vi "Create Event.vi"(3 "error in (no error)":errorcluster, 4 "ExecAnchor in":refnum<class "ExecAnchor.lvclass">) -> (0 "error out":errorcluster, 1 "Event Reg":refnum<event-registration>)   [LabVIEW 2020, in "ExecAnchor.lvclass"]
uses:
  ExecAnchor.lvclass
  ExecAnchor.lvclass/ExecAnchor.ctl
  <vilib>/Utility/error.llb/Error Cluster From Error Code.vi
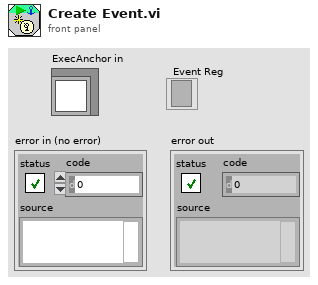
[diagram p1: front panel]
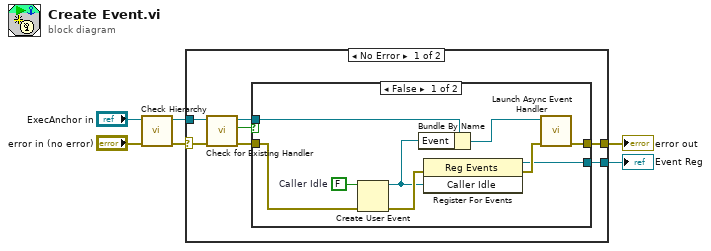
[diagram p0: block diagram]
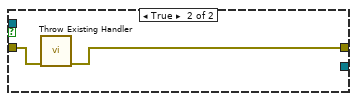
[diagram p2: hidden frame]
diagram:
  n1 = call "Check Hierarchy.vi"("error in (no error)"="error in (no error)", "ExecAnchor in"="ExecAnchor in") -> ("error out"=w2:errorcluster, "ExecAnchor out"=w4:refnum<class "ExecAnchor.lvclass">)  [unwired: 8 in]
  n2 = case shown="No Error" w2 {
    selector: w2 -> [w10 w25]
    tunnel: [w12 _] -> w5
    tunnel: w4 -> [w11 _]
    tunnel: [w13 w25] -> w1
    frame No Error {
      n3 = call "Check for Existing Handler.vi"("error in (no error)"=w10, "ExecAnchor in"=w11) -> ("error out"=w9:errorcluster, "Existing Handler"=w7:bool, "ExecAnchor out"=w8:refnum<class "ExecAnchor.lvclass">)  [unwired: 7 in]
      n4 = case shown="False" w7 {
        tunnel: [w15 w23] -> w13
        tunnel: [w18 _] -> w12
        tunnel: w8 -> [w17 _]
        tunnel: w9 -> [w16 w24]
        frame False {
          w20 = FALSE  # Caller Idle
          n5 = Create User Event(user event datatype=w20, error in=w16) -> (user event=w19:refnum<user-event>, error out=w21:errorcluster)
          n6 = Bundle By Name(cluster=w17, "Event"=w19) -> (w14:refnum<class "ExecAnchor.lvclass">)
          n7 = register-events(error in=w21, w19) -> (reference out=w18:refnum<event-registration>, error out=w22:errorcluster)  [unwired: 1 in]
          n8 = call "Launch Async Event Handler.vi"("error in (no error)"=w22, "ExecAnchor in"=w14) -> ("error out"=w15:errorcluster)  [unwired: 8 in, 1 out]
        }
        frame True {
          n9 = call "Throw Existing Handler.vi"("error in (no error)"=w24) -> ("error out"=w23:errorcluster)  [unwired: 10 in]
        }
      }
    }
    frame Error {
    }
  }
  "error out" <- w1
  "Event Reg" <- w5
